vi "Read Previous Signal Configuration.vi"(8 "error in (no error)":errorcluster, 11 "current signal configuration in":refnum<class "SV Signal.lvclass">) -> (0 "error out":errorcluster, 2 "previous signal configuration":refnum<class "SV Signal.lvclass">, 3 "current signal configuration out":refnum<class "SV Signal.lvclass">)   [LabVIEW 2017, in "SV Signal.lvclass"]
uses:
  <vilib>/addons/_NISVFA/_Generation/Signal Generation/SV Signal/SV Signal.lvclass
  <vilib>/addons/_NISVFA/_Generation/Signal Generation/SV Signal/SV Signal.lvclass/SV Signal.ctl
  <vilib>/addons/_NISVFA/_Generation/Signal Generation/SV Signal/sv_Signal State Attribute.ctl
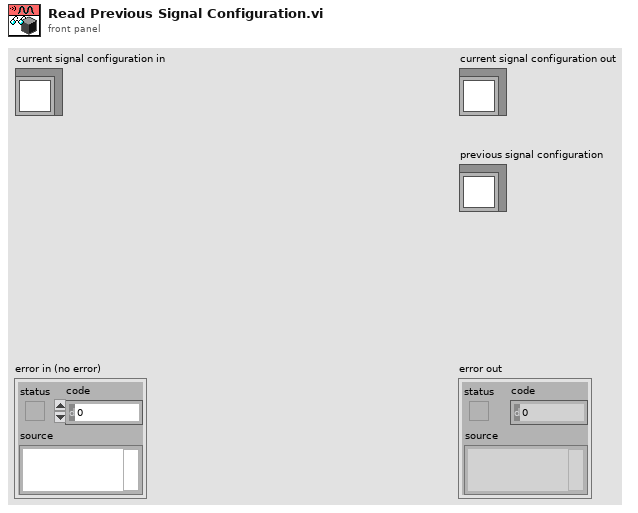
[diagram p1: front panel]
types:
  T1 = typedef "SV Signal.lvclass/sv_Signal State Attribute.ctl" = string
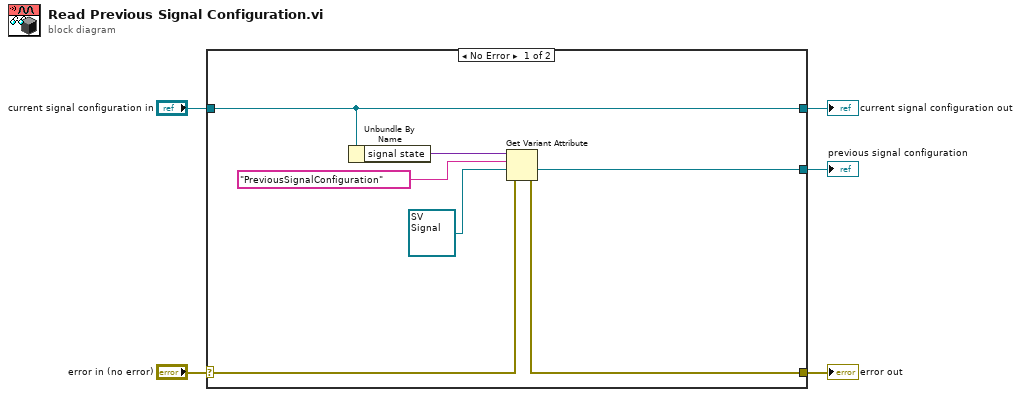
[diagram p0: block diagram]
diagram:
  n1 = case shown="No Error" "error in (no error)" {
    selector: "error in (no error)" -> [w7 w14]
    tunnel: [w6 w14] -> w4
    tunnel: [w12 w13] -> w2
    tunnel: "current signal configuration in" -> [w12 w13]
    tunnel: [w8 _] -> w1
    frame No Error {
      n2 = Unbundle By Name(w12) -> ("signal state"=w11:variant)
      n3 = Get Variant Attribute(Variant=w11, name=T1 "PreviousSignalConfiguration", default value (empty Variant)=refnum<class "SV Signal.lvclass"> refnum ("signal configuration"), error in=w7) -> (value=w8:refnum<class "SV Signal.lvclass">, error out=w6:errorcluster)  [unwired: 2 out]
    }
    frame Error {
    }
  }
  "error out" <- w4
  "current signal configuration out" <- w2
  "previous signal configuration" <- w1
